vi "SetBoolValue.vi"(8 "error in (no error)":errorcluster caption="错误输入（无错误）", 9 "bValue":bool, 10 "strValue":string, 11 "handle":u64) -> (0 "error out":errorcluster caption="错误输出", 2 "function return":i32, 3 "handle out":u64)   [LabVIEW 2011, in "MvCameraControl.lvlib"]
doc: "MV_LV_API int __stdcall SetBoolValue( void* handle, const char* strValue, bool bValue);"
uses:
  MvCameraControl.lvlib
  MvCameraControl.dll
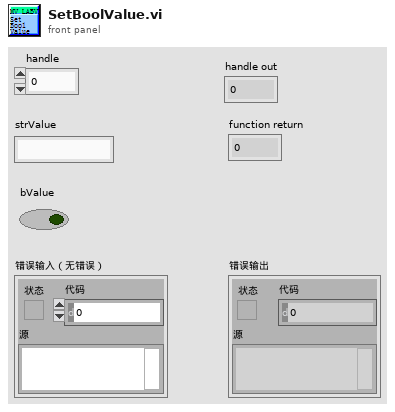
[diagram p1: front panel]
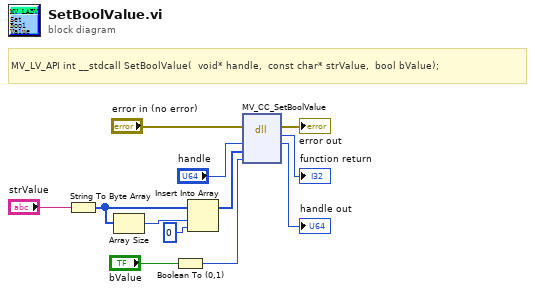
[diagram p0: block diagram]
diagram:
  # "MV_LV_API int __stdcall SetBoolValue(  void* handle,  const char* strValue,  bool bValue);"
  n1 = String To Byte Array(string="strValue") -> (unsigned byte array=w6:u8[])
  n2 = Array Size(array=w6) -> (size(s)=w5:i32)
  n3 = Boolean To (0,1)(Boolean="bValue") -> (0, 1=w9:i16)
  n4 = Insert Into Array(array=w6, index=w5, new element=u8 0 ("新元素/子数组")) -> (w2:u8[])
  n5 = dll-call lib="MvCameraControl.dll" fn="MV_CC_SetBoolValue"(error in="error in (no error)", "handle"="handle", "strKey"=w2, "bValue"=w9) -> (error out=→"error out":errorcluster, "返回类型"=→"function return":i32, "handle"=→"handle out":u64)  [unwired: 4 in, 1 out]
